vi "File.Build Path, Add Multiple Subfolders, Check for invalid Characters.vi"(9 "Check/Create Dir":bool, 10 "Subfolders":string[](array[string]), 11 "Folder":path) -> (0 "error out":errorcluster, 2 "Subfolder":string, 3 "New Path":path)   [LabVIEW 2024]
uses:
  <vilib>/Utility/error.llb/Trim Whitespace One-Sided.vi
  File Utils.lvlib
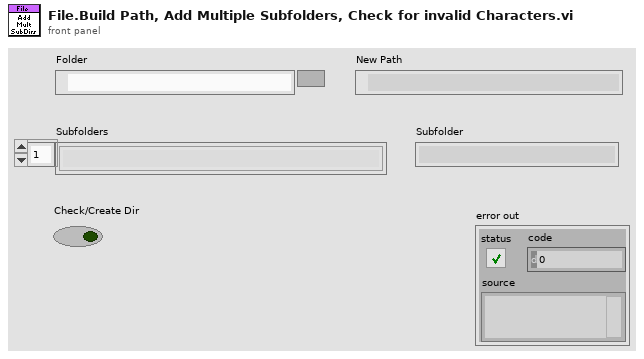
[diagram p1: front panel]
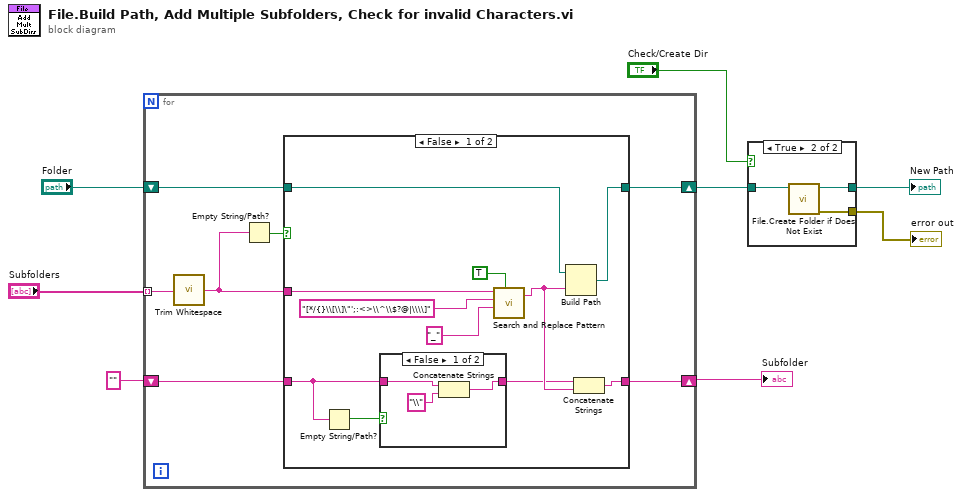
[diagram p0: block diagram]
diagram:
  n1 = for {
    tunnel: "Subfolders" -> [w15] mode=indexing
    shift-right: [w13] -> w6
    shift-left: "Folder" -> [w12]
    shift-right: [w9] -> w1
    shift-left: "" -> [w10]
    n2 = call <vilib>:"Trim Whitespace.vi"("string"=w15) -> ("trimmed string"=w14:string)  [unwired: 1 in]
    n3 = Empty String/Path?(string/path=w14) -> (empty?=w11:bool)
    n4 = case shown="False" w11 {
      tunnel: w14 -> [w25 _]
      tunnel: [w22 w32] -> w13
      tunnel: w12 -> [w21 w32]
      tunnel: w10 -> [w17 w31]
      tunnel: [w19 w31] -> w9
      frame False {
        n5 = Empty String/Path?(string/path=w17) -> (empty?=w18:bool)
        n6 = case shown="False" w18 {
          tunnel: w17 -> [w29 w30]
          tunnel: [w28 w30] -> w16
          frame False {
            n7 = Concatenate Strings(w29, "\\" ("regular expression (\"\")")) -> (w28:string)
          }
          frame True {
          }
        }
        n8 = call <vilib>:"Search and Replace Pattern.vi"("string"=w25, "regular expression (\"\")"="[*/{}\\[\\]\"';:<>\\^\\$?@|\\\\]" ("regular expression (\"\")"), "replace string (\"\")"="_" ("regular expression (\"\")"), "replace all? (F)"=TRUE) -> ("result string"=w20:string)  [unwired: 1 in, 1 out]
        n9 = Build Path(base path=w21, name or relative path=w20) -> (appended path=w22:path)
        n10 = Concatenate Strings(w16, w20) -> (w19:string)
      }
      frame True {
      }
    }
  }
  "Subfolder" <- w1
  n11 = case shown="True" "Check/Create Dir" {
    tunnel: w6 -> [w33 w36]
    tunnel: [w33 w35] -> w5
    tunnel: [_ w34] -> w3
    frame False {
    }
    frame True {
      n12 = call "File.Create Folder if Does Not Exist.vi"("Path"=w36) -> ("error out"=w34:errorcluster, "Dup Path"=w35:path)  [unwired: 8 in, 1 out]
    }
  }
  "New Path" <- w5
  "error out" <- w3
